vi "Set theme path.vi"(8 "error in":errorcluster, 10 "theme path":path, 11 "Theme Config in":refnum<class "Theme Config.lvclass">) -> (0 "error out":errorcluster, 3 "Theme Config out":refnum<class "Theme Config.lvclass">)   [LabVIEW 2021, in "Theme Config.lvclass"]
uses:
  Theme Config.lvclass
  Theme Config.lvclass/Theme Config.ctl
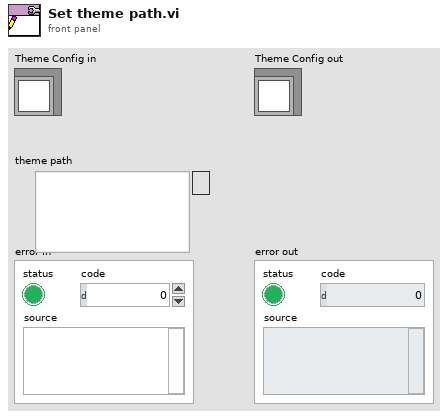
[diagram p1: front panel]
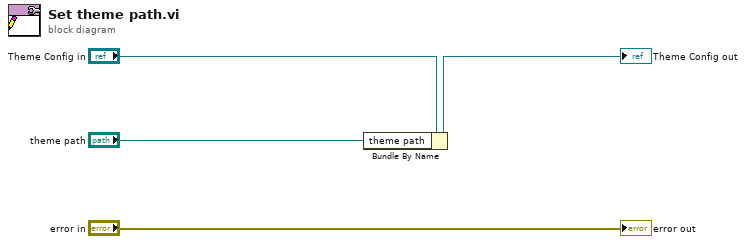
[diagram p0: block diagram]
diagram:
  n1 = Bundle By Name(cluster="Theme Config in", "theme path"="theme path") -> (→"Theme Config out":refnum<class "Theme Config.lvclass">)
  "error out" <- "error in"
